vi "REMOTE RCV.vi"() -> (0 "Buttons Control":T1, 1 "Boolean 2":T2, 2 "Direction 2":T3, 3 "Claw Motor 2":u32(slide) scale=0.0..100.0, 4 "Elbow Motor 2":u32(slide)=50 scale=0.0..100.0, 5 "Shoulder Motor 2":u32(slide)=50 scale=0.0..100.0, 6 "Base Motor 2":u32(slide)=50 scale=0.0..100.0)   [LabVIEW 2015]
uses:
  DIR GAME.ctl
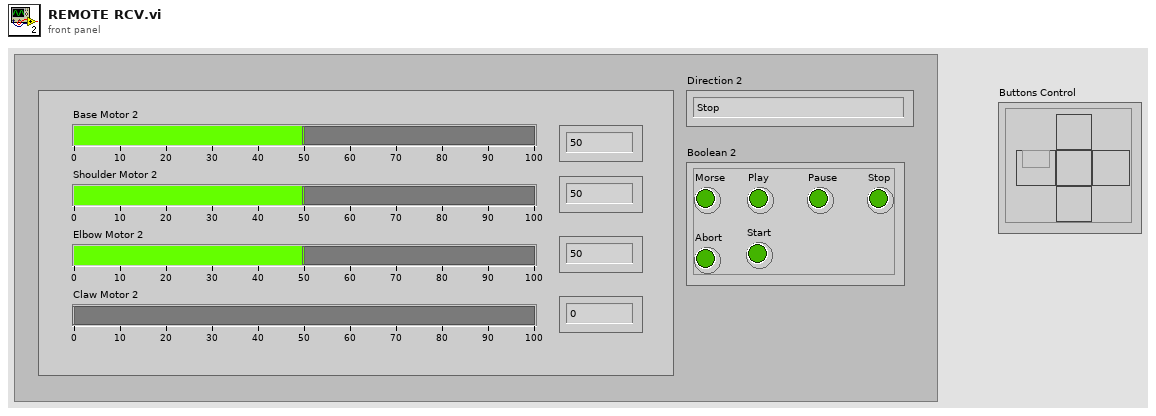
[diagram p1: front panel]
types:
  T1 = cluster{"Front":bool, "Right":bool, "Back":bool, "Left":bool, "Stop":bool}
  T2 = cluster{"Morse":bool, "Play":bool, "Pause":bool, "Stop":bool, "Abort":bool, "Start":bool}
  T3 = typedef "DIR GAME.ctl" = enum16{"Stop", "Front", "FR", "Right", "BR", "Back", "BL", "Left", "FL"}
  T4 = enum16{"Stop", "Front", "FR", "Right", "BR", "Back", "BL", "Left", "FL"}
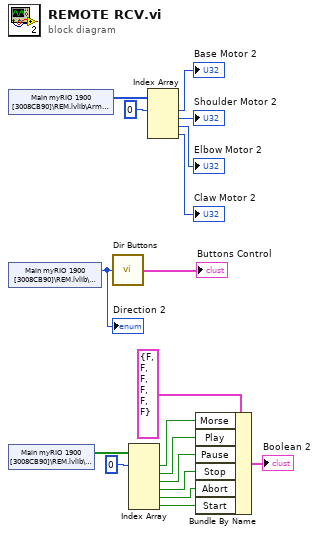
[diagram p0: block diagram]
diagram:
  n1 = shared-variable "Main myRIO 1900 [3008CB90]\\REM.lvlib\\Arm Values"() -> (w18:u32[])  [unwired: 1 in, 1 out]
  n2 = shared-variable "Main myRIO 1900 [3008CB90]\\REM.lvlib\\Direction"() -> (w5:T4)  [unwired: 1 in, 1 out]
  "Direction 2" <- w5
  n3 = shared-variable "Main myRIO 1900 [3008CB90]\\REM.lvlib\\Buttons"() -> (w7:bool[])  [unwired: 1 in, 1 out]
  n4 = call "Dir Buttons.vi"("Direction 2"=w5) -> ("Buttons Control"=→"Buttons Control":T1)
  n5 = Index Array(array=w7, index #1=0 ("index")) -> (element #1=w11:bool, element #2=w10:bool, element #3=w9:bool, element #4=w8:bool, element #5=w6:bool, element #6=w3:bool)  [unwired: 5 in]
  n6 = Index Array(array=w18, index #1=0 ("index")) -> (element #1=→"Base Motor 2":u32, element #2=→"Shoulder Motor 2":u32, element #3=→"Elbow Motor 2":u32, element #4=→"Claw Motor 2":u32)  [unwired: 3 in]
  n7 = Bundle By Name(cluster=T2 {"Morse"=FALSE, "Play"=FALSE, "Pause"=FALSE, "Stop"=FALSE, "Abort"=FALSE, "Start"=FALSE} ("Boolean 3"), "Morse"=w11, "Play"=w10, "Pause"=w9, "Stop"=w8, "Abort"=w6, "Start"=w3) -> (→"Boolean 2":T2)
